vi "Generate HSV colorwheel.vi"(1 "Size":i32=256, 2 "V (intensity)":dbl=255.0 format="%.2f") -> (0 "True-color pixelmap":u32[][](array[numeric]))   [LabVIEW 2022 SP3]
doc: "Author: James Nissen, nissen6@llnl.gov\n\nThis vi generates an HSV color wheel of a particular size and intensity. Use a picture control to display the results."
uses:
  <vilib>/picture/picture.llb/Draw True-Color Pixmap.vi
  <vilib>/Analysis/NI_AALPro.lvlib
panel:
  out "Picture":picture
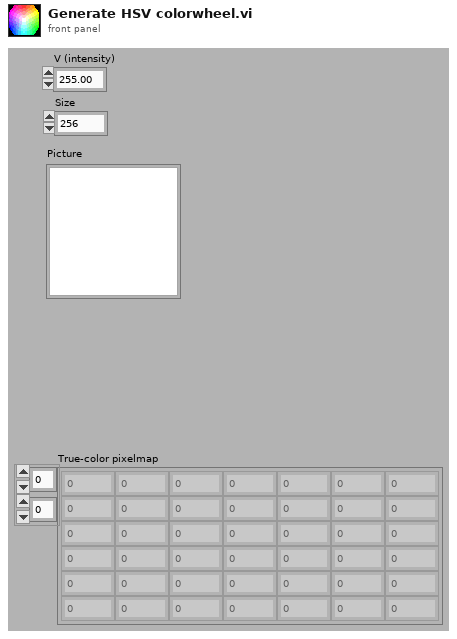
[diagram p1: front panel]
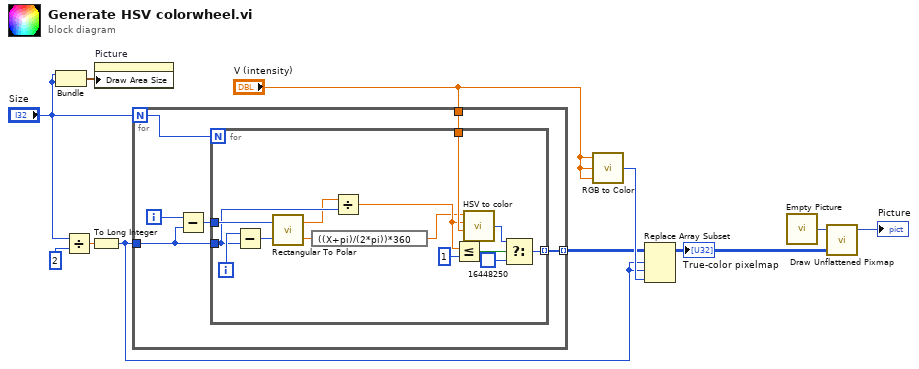
[diagram p0: block diagram]
diagram:
  n1 = Bundle("Size"="Size", "Size"="Size") -> (w1:cluster{"Size":i32, "Size":i32})  [unwired: 1 in]
  n2 = Divide(x="Size", y=2) -> (x/y=w7:dbl)
  n3 = To Long Integer(number=w7) -> (32bit integer=w6:i32)
  n4 = property on="Picture" class="Pict"("Draw Area Size"=w1) -> ()  [unwired: 2 in, 2 out]
  n5 = for {
    N: "Size" -> [w17]
    tunnel: [w15] -> w9 mode=indexing
    tunnel: "V (intensity)" -> [w14]
    tunnel: w6 -> [w12]
    i -> [w13]
    n6 = Subtract(x=w13, y=w12) -> (x-y=w16:i32)
    n7 = for {
      N: w17 -> [_]
      tunnel: w12 -> [w23]
      tunnel: w16 -> [w28]
      tunnel: [w21] -> w15 mode=indexing
      tunnel: w14 -> [w25]
      i -> [w30]
      n8 = Subtract(x=w30, y=w23) -> (x-y=w29:i32)
      n9 = call <vilib>:"Rectangular To Polar.vi"("y"=w29, "x"=w28) -> ("phase"=w19:dbl, "magnitude"=w22:dbl)
      n10 = expression code="((X+pi)/(2*pi))*360"(w19) -> (w18:dbl)
      n11 = Divide(x=w22, y=w23) -> (x/y=w20:dbl)
      n12 = Less Or Equal?(x=w20, y=1) -> (x <= y?=w27:bool)
      n13 = call "HSV to color.vi"("V (intensity)"=w25, "S (Saturation)"=w20, "H (Hue)"=w18) -> ("Color"=w24:u32)  [unwired: 1 in]
      n14 = Select(t=w24, s=w27, f=u32 16448250) -> (s? t:f=w21:u32)
    }
  }
  n15 = call <vilib>:"RGB to Color.vi"("B"="V (intensity)", "G"="V (intensity)", "R"="V (intensity)") -> ("Color"=w10:u32)
  n16 = Replace Array Subset(array=w9, new element=w10, index (row)=w6, index (col)=w6) -> (w5:u32[][])
  "True-color pixelmap" <- w5
  n17 = call "Empty Picture"() -> ("empty picture"=w4:picture)
  n18 = call-poly <vilib>:"Draw Unflattened Pixmap.vi"("picture"=w4, "data (RGB format)"=w5) -> ("new picture"=→"Picture":picture)  [unwired: 7 in]
